vi "Get ni-xnet ports.vi"(8 "Error In":errorcluster, 11 "Device Item Ref in":T1 format="%.0x") -> (0 "Error Out":errorcluster, 1 "NI-XNET Port Item Paths":string[](array[string]), 2 "NI-XNET Port Refs":T1[](array[typedef]) format="%.0x", 3 "Device Item Ref out":T1 format="%.0x")   [LabVIEW 2018, in "NI-XNET Monitor System Explorer.lvlib"]
uses:
  NI-XNET Monitor System Explorer.lvlib
  <vilib>/NI Veristand/Custom Device API/Custom Device Item Ref.ctl
  Shared/Constants.vi
  <vilib>/NI Veristand/Custom Device Tools/Custom Device Utility Library/NI VeriStand - Search for Item by GUID.vi
  <vilib>/NI Veristand/Custom Device Tools/Custom Device Utility Library/Custom Device Utility Library.lvlib
  Shared/NI-XNET Monitor Shared.lvlib
  <vilib>/NI Veristand/Custom Device API/Custom Device API.lvlib
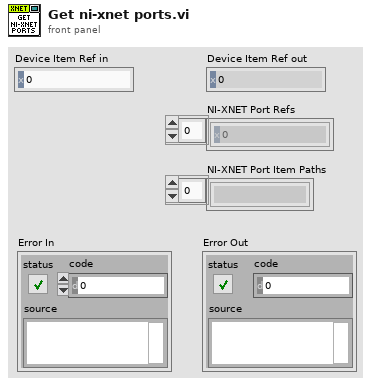
[diagram p1: front panel]
types:
  T1 = typedef "Custom Device API.lvlib/Custom Device Item Ref.ctl" = u64
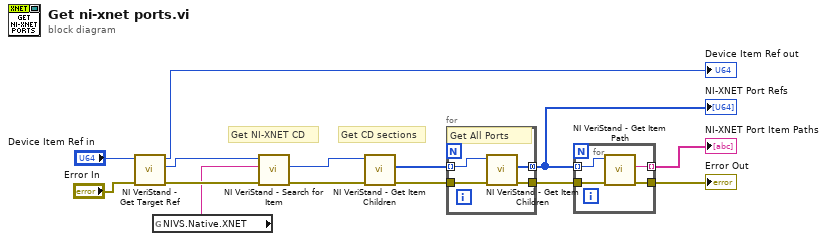
[diagram p0: block diagram]
diagram:
  # "Get CD sections"
  # "Get NI-XNET CD"
  n1 = call <vilib>:"NI VeriStand - Get Target Ref.vi"("error in"="Error In", "Item Ref in"="Device Item Ref in") -> ("error out"=w11:errorcluster, "Target Ref"=w6:T1, "Item Ref out"=→"Device Item Ref out":T1)  [unwired: 6 in, 1 out]
  n2 = global read "Constants.vi" "NIVS.Native.XNET"() -> (w7:string)
  n3 = call-poly <vilib>:"NI VeriStand - Search for Item.vi"("error in"=w11, "Item GUID"=w7, "Section Ref in"=w6) -> ("error out"=w10:errorcluster, "Item Ref"=w8:T1)  [unwired: 5 in, 2 out]
  n4 = call <vilib>:"NI VeriStand - Get Item Children.vi"("error in (no error)"=w10, "Item Ref in"=w8) -> ("error out"=w12:errorcluster, "Child Refs"=w9:T1[])  [unwired: 6 in, 2 out]
  n5 = for {
    tunnel: w9 -> [w16] mode=indexing
    tunnel: w12 -> [w15]
    tunnel: [w18] -> w1 mode=concatenating
    tunnel: [w17] -> w4
    # "Get All Ports"
    n6 = call <vilib>:"NI VeriStand - Get Item Children.vi"("error in (no error)"=w15, "Item Ref in"=w16) -> ("error out"=w17:errorcluster, "Child Refs"=w18:T1[])  [unwired: 6 in, 2 out]
  }
  "NI-XNET Port Refs" <- w1
  n7 = for {
    tunnel: w1 -> [w22] mode=indexing
    tunnel: w4 -> [w21]
    tunnel: [w20] -> w3
    tunnel: [w19] -> w2 mode=indexing
    n8 = call <vilib>:"NI VeriStand - Get Item Path.vi"("error in (no error)"=w21, "Item Ref in"=w22) -> ("error out"=w20:errorcluster, "Path"=w19:string)  [unwired: 6 in, 2 out]
  }
  "Error Out" <- w3
  "NI-XNET Port Item Paths" <- w2
